vi "read Txt Files.vi"(10 "file path (use dialog)":path) -> (1 "error out":errorcluster, 2 "number":T1)   [LabVIEW 2017] (continued)
Position(0.1mm)¡G\t0.000000\tVelocity(0.1mm0/s)¡G\t0.000000\tVoltage¡G\t-0.009460\nReal Periold(ms)¡G\t1\tEncoder Position(0.1mm)¡G\t0.000000\tVelocity(0.1mm0/s)¡G\t0.000000\tVoltage¡G\t-0.001801\nReal Periold(ms)¡G\t1\tEncoder Position(0.1mm)¡G\t0.000000\tVelocity(0.1mm0/s)¡G\t0.000000\tVoltage¡G\t0.034485\nReal Periold(ms)¡G\t1\tEncoder Position(0.1mm)¡G\t0.000000\tVelocity(0.1mm0/s)¡G\t0.000000\tVoltage¡G\t-0.005951\nReal Periold(ms)¡G\t1\tEncoder Position(0.1mm)¡G\t0.000000\tVelocity(0.1mm0/s)¡G\t0.000000\tVoltage¡G\t0.003601\nReal Periold(ms)¡G\t1\tEncoder Position(0.1mm)¡G\t0.000000\tVelocity(0.1mm0/s)¡G\t0.000000\tVoltage¡G\t0.002319\nReal Periold(ms)¡G\t1\tEncoder Position(0.1mm)¡G\t0.000000\tVelocity(0.1mm0/s)¡G\t0.000000\tVoltage¡G\t0.000092\nReal Periold(ms)¡G\t1\tEncoder Position(0.1mm)¡G\t0.000000\tVelocity(0.1mm0/s)¡G\t0.000000\tVoltage¡G\t0.002960\nReal Periold(ms)¡G\t1\tEncoder Position(0.1mm)¡G\t0.000000\tVelocity(0.1mm0/s)¡G\t0.000000\tVoltage¡G\t0.002319\nReal Periold(ms)¡G\t1\tEncoder Position(0.1mm)¡G\t0.000000\tVelocity(0.1mm0/s)¡G\t0.000000\tVoltage¡G\t0.004883\nReal Periold(ms)¡G\t1\tEncoder Position(0.1mm)¡G\t0.000000\tVelocity(0.1mm0/s)¡G\t0.000000\tVoltage¡G\t-0.004669\nReal Periold(ms)¡G\t1\tEncoder Position(0.1mm)¡G\t0.000000\tVelocity(0.1mm0/s)¡G\t0.000000\tVoltage¡G\t-0.003723\nReal Periold(ms)¡G\t1\tEncoder Position(0.1mm)¡G\t0.000000\tVelocity(0.1mm0/s)¡G\t0.000000\tVoltage¡G\t0.004883\nReal Periold(ms)¡G\t1\tEncoder Position(0.1mm)¡G\t0.000000\tVelocity(0.1mm0/s)¡G\t0.000000\tVoltage¡G\t-0.007843\nReal Periold(ms)¡G\t1\tEncoder Position(0.1mm)¡G\t0.000000\tVelocity(0.1mm0/s)¡G\t0.000000\tVoltage¡G\t-0.005951\nReal Periold(ms)¡G\t1\tEncoder Position(0.1mm)¡G\t0.000000\tVelocity(0.1mm0/s)¡G\t0.000000\tVoltage¡G\t-0.007538\nReal Periold(ms)¡G\t1\tEncoder Position(0.1mm)¡G\t0.000000\tVelocity(0.1mm0/s)¡G\t0.000000\tVoltage¡G\t-0.001495\nReal Periold(ms)¡G\t1\tEncoder Position(0.1mm)¡G\t0.000000\tVelocity(0.1mm0/s)¡G\t0.000000\tVoltage¡G\t-0.001801\nReal Periold(ms)¡G\t1\tEncoder Position(0.1mm)¡G\t0.000000\tVelocity(0.1mm0/s)¡G\t0.000000\tVoltage¡G\t-0.006592\nReal Periold(ms)¡G\t1\tEncoder Position(0.1mm)¡G\t0.000000\tVelocity(0.1mm0/s)¡G\t0.000000\tVoltage¡G\t0.002655\nReal Periold(ms)¡G\t1\tEncoder Position(0.1mm)¡G\t0.000000\tVelocity(0.1mm0/s)¡G\t0.000000\tVoltage¡G\t-0.007843\nReal Periold(ms)¡G\t1\tEncoder Position(0.1mm)¡G\t0.000000\tVelocity(0.1mm0/s)¡G\t0.000000\tVoltage¡G\t-0.007538\nReal Periold(ms)¡G\t1\tEncoder Position(0.1mm)¡G\t0.000000\tVelocity(0.1mm0/s)¡G\t0.000000\tVoltage¡G\t0.006775\nReal Periold(ms)¡G\t1\tEncoder Position(0.1mm)¡G\t0.000000\tVelocity(0.1mm0/s)¡G\t0.000000\tVoltage¡G\t0.005188\nReal Periold(ms)¡G\t1\tEncoder Position(0.1mm)¡G\t0.000000\tVelocity(0.1mm0/s)¡G\t0.000000\tVoltage¡G\t-0.068329\nReal Periold(ms)¡G\t1\tEncoder Position(0.1mm)¡G\t0.000000\tVelocity(0.1mm0/s)¡G\t0.000000\tVoltage¡G\t0.000732\nReal Periold(ms)¡G\t1\tEncoder Position(0.1mm)¡G\t0.000000\tVelocity(0.1mm0/s)¡G\t0.000000\tVoltage¡G\t0.002014\nReal Periold(ms)¡G\t1\tEncoder Position(0.1mm)¡G\t0.000000\tVelocity(0.1mm0/s)¡G\t0.000000\tVoltage¡G\t-0.003082\nReal Periold(ms)¡G\t1\tEncoder Position(0.1mm)¡G\t0.000000\tVelocity(0.1mm0/s)¡G\t0.000000\tVoltage¡G\t-0.022827\nReal Periold(ms)¡G\t1\tEncoder Position(0.1mm)¡G\t0.000000\tVelocity(0.1mm0/s)¡G\t0.000000\tVoltage¡G\t0.007416\nReal Periold(ms)¡G\t1\tEncoder Position(0.1mm)¡G\t0.000000\tVelocity(0.1mm0/s)¡G\t0.000000\tVoltage¡G\t-0.004028\nReal Periold(ms)¡G\t1\tEncoder Position(0.1mm)¡G\t0.000000\tVelocity(0.1mm0/s)¡G\t0.000000\tVoltage¡G\t-0.002441\nReal Periold(ms)¡G\t1\tEncoder Position(0.1mm)¡G\t0.000000\tVelocity(0.1mm0/s)¡G\t0.000000\tVoltage¡G\t-0.001160\nReal Periold(ms)¡G\t1\tEncoder Position(0.1mm)¡G\t0.000000\tVelocity(0.1mm0/s)¡G\t0.000000\tVoltage¡G\t0.000427\nReal Periold(ms)¡G\t1\tEncoder Position(0.1mm)¡G\t0.000000\tVelocity(0.1mm0/s)¡G\t0.000000\tVoltage¡G\t-0.012299\nReal Periold(ms)¡G\t1\tEncoder Position(0.1mm)¡G\t0.000000\tVelocity(0.1mm0/s)¡G\t0.000000\tVoltage¡G\t0.007111\nReal Periold(ms)¡G\t1\tEncoder Position(0.1mm)¡G\t0.000000\tVelocity(0.1mm0/s)¡G\t0.000000\tVoltage¡G\t-0.057831\nReal Periold(ms)¡G\t1\tEncoder Position(0.1mm)¡G\t0.000000\tVelocity(0.1mm0/s)¡G\t0.000000\tVoltage¡G\t0.005524\nReal Periold(ms)¡G\t1\tEncoder Position(0.1mm)¡G\t0.000000\tVelocity(0.1mm0/s)¡G\t0.000000\tVoltage¡G\t-0.004669\nReal Periold(ms)¡G\t1\tEncoder Position(0.1mm)¡G\t0.000000\tVelocity(0.1mm0/s)¡G\t0.000000\tVoltage¡G\t-0.002777\nReal Periold(ms)¡G\t1\tEncoder Position(0.1mm)¡G\t0.000000\tVelocity(0.1mm0/s)¡G\t0.000000\tVoltage¡G\t-0.005005\nReal Periold(ms)¡G\t1\tEncoder Position(0.1mm)¡G\t0.000000\tVelocity(0.1mm0/s)¡G\t0.000000\tVoltage¡G\t-0.005005\nReal Periold(ms)¡G\t1\tEncoder Position(0.1mm)¡G\t0.000000\tVelocity(0.1mm0/s)¡G\t0.000000\tVoltage¡G\t0.010284\nReal Periold(ms)¡G\t1\tEncoder Position(0.1mm)¡G\t0.000000\tVelocity(0.1mm0/s)¡G\t0.000000\tVoltage¡G\t-0.002777\nReal Periold(ms)¡G\t1\tEncoder Position(0.1mm)¡G\t0.000000\tVelocity(0.1mm0/s)¡G\t0.000000\tVoltage¡G\t-0.010071\nReal Periold(ms)¡G\t1\tEncoder Position(0.1mm)¡G\t0.000000\tVelocity(0.1mm0/s)¡G\t0.000000\tVoltage¡G\t0.001373\nReal Periold(ms)¡G\t1\tEncoder Position(0.1mm)¡G\t0.000000\tVelocity(0.1mm0/s)¡G\t0.000000\tVoltage¡G\t-0.001801\nReal Periold(ms)¡G\t1\tEncoder Position(0.1mm)¡G\t0.000000\tVelocity(0.1mm0/s)¡G\t0.000000\tVoltage¡G\t-0.003723\nReal Periold(ms)¡G\t1\tEncoder Position(0.1mm)¡G\t0.000000\tVelocity(0.1mm0/s)¡G\t0.000000\tVoltage¡G\t0.010590\nReal Periold(ms)¡G\t1\tEncoder Position(0.1mm)¡G\t0.000000\tVelocity(0.1mm0/s)¡G\t0.000000\tVoltage¡G\t0.002014\nReal Periold(ms)¡G\t1\tEncoder Position(0.1mm)¡G\t0.000000\tVelocity(0.1mm0/s)¡G\t0.000000\tVoltage¡G\t-0.005310\nReal Periold(ms)¡G\t1\tEncoder Position(0.1mm)¡G\t0.000000\tVelocity(0.1mm0/s)¡G\t0.000000\tVoltage¡G\t0.002655\nReal Periold(ms)¡G\t1\tEncoder Position(0.1mm)¡G\t0.000000\tVelocity(0.1mm0/s)¡G\t0.000000\tVoltage¡G\t-0.011353\nReal Periold(ms)¡G\t1\tEncoder Position(0.1mm)¡G\t0.000000\tVelocity(0.1mm0/s)¡G\t0.000000\tVoltage¡G\t0.001068\nReal Periold(ms)¡G\t1\tEncoder Position(0.1mm)¡G\t0.000000\tVelocity(0.1mm0/s)¡G\t0.000000\tVoltage¡G\t-0.002136\nReal Periold(ms)¡G\t1\tEncoder Position(0.1mm)¡G\t0.000000\tVelocity(0.1mm0/s)¡G\t0.000000\tVoltage¡G\t-0.003387\nReal Periold(ms)¡G\t1\tEncoder Position(0.1mm)¡G\t0.000000\tVelocity(0.1mm0/s)¡G\t0.000000\tVoltage¡G\t0.003601\nReal Periold(ms)¡G\t1\tEncoder Position(0.1mm)¡G\t0.000000\tVelocity(0.1mm0/s)¡G\t0.000000\tVoltage¡G\t0.001068\nReal Periold(ms)¡G\t1\tEncoder Position(0.1mm)¡G\t0.000000\tVelocity(0.1mm0/s)¡G\t0.000000\tVoltage¡G\t-0.005005\nReal Periold(ms)¡G\t1\tEncoder Position(0.1mm)¡G\t0.000000\tVelocity(0.1mm0/s)¡G\t0.000000\tVoltage¡G\t-0.014526\nReal Periold(ms)¡G\t1\tEncoder Position(0.1mm)¡G\t0.000000\tVelocity(0.1mm0/s)¡G\t0.000000\tVoltage¡G\t0.005188\nReal Periold(ms)¡G\t1\tEncoder Position(0.1mm)¡G\t0.000000\tVelocity(0.1mm0/s)¡G\t0.000000\tVoltage¡G\t-0.000214\nReal Periold(ms)¡G\t1\tEncoder Position(0.1mm)¡G\t0.000000\tVelocity(0.1mm0/s)¡G\t0.000000\tVoltage¡G\t-0.002136\nReal Periold(ms)¡G\t1\tEncoder Position(0.1mm)¡G\t0.000000\tVelocity(0.1mm0/s)¡G\t0.000000\tVoltage¡G\t-0.005310\nReal Periold(ms)¡G\t1\tEncoder Position(0.1mm)¡G\t0.000000\tVelocity(0.1mm0/s)¡G\t0.000000\tVoltage¡G\t-0.002777\nReal Periold(ms)¡G\t1\tEncoder Position(0.1mm)¡G\t0.000000\tVelocity(0.1mm0/s)¡G\t0.000000\tVoltage¡G\t0.001373\nReal Periold(ms)¡G\t1\tEncoder Position(0.1mm)¡G\t0.000000\tVelocity(0.1mm0/s)¡G\t0.000000\tVoltage¡G\t-0.013580\nReal Periold(ms)¡G\t1\tEncoder Position(0.1mm)¡G\t0.000000\tVelocity(0.1mm0/s)¡G\t0.000000\tVoltage¡G\t-0.009460\nReal Periold(ms)¡G\t1\tEncoder Position(0.1mm)¡G\t0.000000\tVelocity(0.1mm0/s)¡G\t0.000000\tVoltage¡G\t-0.002441\nReal Periold(ms)¡G\t1\tEncoder Position(0.1mm)¡G\t0.000000\tVelocity(0.1mm0/s)¡G\t0.000000\tVoltage¡G\t0.011230\nReal Periold(ms)¡G\t1\tEncoder Position(0.1mm)¡G\t0.000000\tVelocity(0.1mm0/s)¡G\t0.000000\tVoltage¡G\t-0.005951\nReal Periold(ms)¡G\t1\tEncoder Position(0.1mm)¡G\t0.000000\tVelocity(0.1mm0/s)¡G\t0.000000\tVoltage¡G\t0.008362\nReal Periold(ms)¡G\t1\tEncoder Position(0.1mm)¡G\t0.000000\tVelocity(0.1mm0/s)¡G\t0.000000\tVoltage¡G\t0.009979\nReal Periold(ms)¡G\t1\tEncoder Position(0.1mm)¡G\t0.000000\tVelocity(0.1mm0/s)¡G\t0.000000\tVoltage¡G\t-0.008179\nReal Periold(ms)¡G\t1\tEncoder Position(0.1mm)¡G\t0.000000\tVelocity(0.1mm0/s)¡G\t0.000000\tVoltage¡G\t-0.003723\nReal Periold(ms)¡G\t1\tEncoder Position(0.1mm)¡G\t0.000000\tVelocity(0.1mm0/s)¡G\t0.000000\tVoltage¡G\t0.008362\nReal Periold(ms)¡G\t1\tEncoder Position(0.1mm)¡G\t0.000000\tVelocity(0.1mm0/s)¡G\t0.000000\tVoltage¡G\t-0.001801\nReal Periold(ms)¡G\t1\tEncoder Position(0.1mm)¡G\t0.000000\tVelocity(0.1mm0/s)¡G\t0.000000\tVoltage¡G\t0.000092\nReal Periold(ms)¡G\t1\tEncoder Position(0.1mm)¡G\t0.000000\tVelocity(0.1mm0/s)¡G\t0.000000\tVoltage¡G\t-0.005951\nReal Periold(ms)¡G\t1\tEncoder Position(0.1mm)¡G\t0.000000\tVelocity(0.1mm0/s)¡G\t0.000000\tVoltage¡G\t-0.014221\nReal Periold(ms)¡G\t1\tEncoder Position(0.1mm)¡G\t0.000000\tVelocity(0.1mm0/s)¡G\t0.000000\tVoltage¡G\t-0.005005\nReal Periold(ms)¡G\t1\tEncoder Position(0.1mm)¡G\t0.000000\tVelocity(0.1mm0/s)¡G\t0.000000\tVoltage¡G\t0.050720\nReal Periold(ms)¡G\t1\tEncoder Position(0.1mm)¡G\t0.000000\tVelocity(0.1mm0/s)¡G\t0.000000\tVoltage¡G\t0.006775\nReal Periold(ms)¡G\t1\tEncoder Position(0.1mm)¡G\t0.000000\tVelocity(0.1mm0/s)¡G\t0.000000\tVoltage¡G\t-0.003387\nReal Periold(ms)¡G\t1\tEncoder Position(0.1mm)¡G\t0.000000\tVelocity(0.1mm0/s)¡G\t0.000000\tVoltage¡G\t0.003601\nReal Periold(ms)¡G\t1\tEncoder Position(0.1mm)¡G\t0.000000\tVelocity(0.1mm0/s)¡G\t0.000000\tVoltage¡G\t0.000092\nReal Periold(ms)¡G\t1\tEncoder Position(0.1mm)¡G\t0.000000\tVelocity(0.1mm0/s)¡G\t0.000000\tVoltage¡G\t-0.000854\nReal Periold(ms)¡G\t1\tEncoder Position(0.1mm)¡G\t0.000000\tVelocity(0.1mm0/s)¡G\t0.000000\tVoltage¡G\t-0.004028\nReal Periold(ms)¡G\t1\tEncoder Position(0.1mm)¡G\t0.000000\tVelocity(0.1mm0/s)¡G\t0.000000\tVoltage¡G\t0.000427\nReal Periold(ms)¡G\t1\tEncoder Position(0.1mm)¡G\t0.000000\tVelocity(0.1mm0/s)¡G\t0.000000\tVoltage¡G\t0.002655\nReal Periold(ms)¡G\t1\tEncoder Position(0.1mm)¡G\t0.000000\tVelocity(0.1mm0/s)¡G\t0.000000\tVoltage¡G\t-0.007843\nReal Periold(ms)¡G\t1\tEncoder Position(0.1mm)¡G\t0.000000\tVelocity(0.1mm0/s)¡G\t0.000000\tVoltage¡G\t0.000092\nReal Periold(ms)¡G\t1\tEncoder Position(0.1mm)¡G\t0.000000\tVelocity(0.1mm0/s)¡G\t0.000000\tVoltage¡G\t-0.009125\nReal Periold(ms)¡G\t1\tEncoder Position(0.1mm)¡G\t0.000000\tVelocity(0.1mm0/s)¡G\t0.000000\tVoltage¡G\t0.010284\nReal Periold(ms)¡G\t1\tEncoder Position(0.1mm)¡G\t0.000000\tVelocity(0.1mm0/s)¡G\t0.000000\tVoltage¡G\t0.002960\nReal Periold(ms)¡G\t1\tEncoder Position(0.1mm)¡G\t0.000000\tVelocity(0.1mm0/s)¡G\t0.000000\tVoltage¡G\t0.002960\nReal Periold(ms)¡G\t1\tEncoder Position(0.1mm)¡G\t0.000000\tVelocity(0.1mm0/s)¡G\t0.000000\tVoltage¡G\t0.007751\nReal Periold(ms)¡G\t1\tEncoder Position(0.1mm)¡G\t0.000000\tVelocity(0.1mm0/s)¡G\t0.000000\tVoltage¡G\t0.008057\nReal Periold(ms)¡G\t1\tEncoder Position(0.1mm)¡G\t0.000000\tVelocity(0.1mm0/s)¡G\t0.000000\tVoltage¡G\t-0.000214\nReal Periold(ms)¡G\t1\tEncoder Position(0.1mm)¡G\t0.000000\tVelocity(0.1mm0/s)¡G\t0.000000\tVoltage¡G\t-0.004028\nReal Periold(ms)¡G\t1\tEncoder Position(0.1mm)¡G\t0.000000\tVelocity(0.1mm0/s)¡G\t0.000000\tVoltage¡G\t-0.003723\nReal Periold(ms)¡G\t1\tEncoder Position(0.1mm)¡G\t0.000000\tVelocity(0.1mm0/s)¡G\t0.000000\tVoltage¡G\t-0.002777\nReal Periold(ms)¡G\t1\tEncoder Position(0.1mm)¡G\t0.000000\tVelocity(0.1mm0/s)¡G\t0.000000\tVoltage¡G\t-0.008179\nReal Periold(ms)¡G\t1\tEncoder Position(0.1mm)¡G\t0.000000\tVelocity(0.1mm0/s)¡G\t0.000000\tVoltage¡G\t-0.010712\nReal Periold(ms)¡G\t1\tEncoder Position(0.1mm)¡G\t0.000000\tVelocity(0.1mm0/s)¡G\t0.000000\tVoltage¡G\t-0.002136\nReal Periold(ms)¡G\t1\tEncoder Position(0.1mm)¡G\t0.000000\tVelocity(0.1mm0/s)¡G\t0.000000\tVoltage¡G\t-0.011353\nReal Periold(ms)¡G\t1\tEncoder Position(0.1mm)¡G\t0.000000\tVelocity(0.1mm0/s)¡G\t0.000000\tVoltage¡G\t0.000092\nReal Periold(ms)¡G\t1\tEncoder Position(0.1mm)¡G\t0.000000\tVelocity(0.1mm0/s)¡G\t0.000000\tVoltage¡G\t0.010590\nReal Periold(ms)¡G\t1\tEncoder Position(0.1mm)¡G\t0.000000\tVelocity(0.1mm0/s)¡G\t0.000000\tVoltage¡G\t-0.023773\nReal Periold(ms)¡G\t1\tEncoder Position(0.1mm)¡G\t0.000000\tVelocity(0.1mm0/s)¡G\t0.000000\tVoltage¡G\t-0.005951\nReal Periold(ms)¡G\t1\tEncoder Position(0.1mm)¡G\t0.000000\tVelocity(0.1mm0/s)¡G\t0.000000\tVoltage¡G\t0.005188\nReal Periold(ms)¡G\t1\tEncoder Position(0.1mm)¡G\t0.000000\tVelocity(0.1mm0/s)¡G\t0.000000\tVoltage¡G\t0.000092\nReal Periold(ms)¡G\t1\tEncoder Position(0.1mm)¡G\t0.000000\tVelocity(0.1mm0/s)¡G\t0.000000\tVoltage¡G\t0.010284\nReal Periold(ms)¡G\t1\tEncoder Position(0.1mm)¡G\t0.000000\tVelocity(0.1mm0/s)¡G\t0.000000\tVoltage¡G\t0.004547\nReal Periold(ms)¡G\t1\tEncoder Position(0.1mm)¡G\t0.000000\tVelocity(0.1mm0/s)¡G\t0.000000\tVoltage¡G\t-0.004364\nReal Periold(ms)¡G\t1\tEncoder Position(0.1mm)¡G\t0.000000\tVelocity(0.1mm0/s)¡G\t0.000000\tVoltage¡G\t0.000092\nReal Periold(ms)¡G\t1\tEncoder Position(0.1mm)¡G\t0.000000\tVelocity(0.1mm0/s)¡G\t0.000000\tVoltage¡G\t-0.010071\nReal Periold(ms)¡G\t1\tEncoder Position(0.1mm)¡G\t0.000000\tVelocity(0.1mm0/s)¡G\t0.000000\tVoltage¡G\t-0.002136\nReal Periold(ms)¡G\t1\tEncoder Position(0.1mm)¡G\t0.000000\tVelocity(0.1mm0/s)¡G\t0.000000\tVoltage¡G\t-0.012634\nReal Periold(ms)¡G\t1\tEncoder Position(0.1mm)¡G\t0.000000\tVelocity(0.1mm0/s)¡G\t0.000000\tVoltage¡G\t0.002960\nReal Periold(ms)¡G\t1\tEncoder Position(0.1mm)¡G\t0.000000\tVelocity(0.1mm0/s)¡G\t0.000000\tVoltage¡G\t-0.013275\nReal Periold(ms)¡G\t1\tEncoder Position(0.1mm)¡G\t0.000000\tVelocity(0.1mm0/s)¡G\t0.000000\tVoltage¡G\t-0.007233\nReal Periold(ms)¡G\t1\tEncoder Position(0.1mm)¡G\t0.000000\tVelocity(0.1mm0/s)¡G\t0.000000\tVoltage¡G\t-0.001495\nReal Periold(ms)¡G\t1\tEncoder Position(0.1mm)¡G\t0.000000\tVelocity(0.1mm0/s)¡G\t0.000000\tVoltage¡G\t0.007111\nReal Periold(ms)¡G\t1\tEncoder Position(0.1mm)¡G\t0.000000\tVelocity(0.1mm0/s)¡G\t0.000000\tVoltage¡G\t-0.004364\nReal Periold(ms)¡G\t1\tEncoder Position(0.1mm)¡G\t0.000000\tVelocity(0.1mm0/s)¡G\t0.000000\tVoltage¡G\t0.000092\nReal Periold(ms)¡G\t1\tEncoder Position(0.1mm)¡G\t0.000000\tVelocity(0.1mm0/s)¡G\t0.000000\tVoltage¡G\t0.024292\nReal Periold(ms)¡G\t1\tEncoder Position(0.1mm)¡G\t0.000000\tVelocity(0.1mm0/s)¡G\t0.000000\tVoltage¡G\t-0.019318\nReal Periold(ms)¡G\t1\tEncoder Position(0.1mm)¡G\t0.000000\tVelocity(0.1mm0/s)¡G\t0.000000\tVoltage¡G\t-0.028870\nReal Periold(ms)¡G\t1\tEncoder Position(0.1mm)¡G\t0.000000\tVelocity(0.1mm0/s)¡G\t0.000000\tVoltage¡G\t-0.002441\nReal Periold(ms)¡G\t1\tEncoder Position(0.1mm)¡G\t0.000000\tVelocity(0.1mm0/s)¡G\t0.000000\tVoltage¡G\t-0.003082\nReal Periold(ms)¡G\t1\tEncoder Position(0.1mm)¡G\t0.000000\tVelocity(0.1mm0/s)¡G\t0.000000\tVoltage¡G\t-0.011688\nReal Periold(ms)¡G\t1\tEncoder Position(0.1mm)¡G\t0.000000\tVelocity(0.1mm0/s)¡G\t0.000000\tVoltage¡G\t0.008698\nReal Periold(ms)¡G\t1\tEncoder Position(0.1mm)¡G\t0.000000\tVelocity(0.1mm0/s)¡G\t0.000000\tVoltage¡G\t-0.003082\nReal Periold(ms)¡G\t1\tEncoder Position(0.1mm)¡G\t0.000000\tVelocity(0.1mm0/s)¡G\t0.000000\tVoltage¡G\t0.017914\nReal Periold(ms)¡G\t1\tEncoder Position(0.1mm)¡G\t0.000000\tVelocity(0.1mm0/s)¡G\t0.000000\tVoltage¡G\t-0.018677\nReal Periold(ms)¡G\t1\tEncoder Position(0.1mm)¡G\t0.000000\tVelocity(0.1mm0/s)¡G\t0.000000\tVoltage¡G\t-0.008179\nReal Periold(ms)¡G\t1\tEncoder Position(0.1mm)¡G\t0.000000\tVelocity(0.1mm0/s)¡G\t0.000000\tVoltage¡G\t-0.009766\nReal Periold(ms)¡G\t1\tEncoder Position(0.1mm)¡G\t0.000000\tVelocity(0.1mm0/s)¡G\t0.000000\tVoltage¡G\t-0.004364\nReal Periold(ms)¡G\t1\tEncoder Position(0.1mm)¡G\t0.000000\tVelocity(0.1mm0/s)¡G\t0.000000\tVoltage¡G\t-0.004669\nReal Periold(ms)¡G\t1\tEncoder Position(0.1mm)¡G\t0.000000\tVelocity(0.1mm0/s)¡G\t0.000000\tVoltage¡G\t0.012207\nReal Periold(ms)¡G\t1\tEncoder Position(0.1mm)¡G\t0.000000\tVelocity(0.1mm0/s)¡G\t0.000000\tVoltage¡G\t0.013153\nReal Periold(ms)¡G\t1\tEncoder Position(0.1mm)¡G\t0.000000\tVelocity(0.1mm0/s)¡G\t0.000000\tVoltage¡G\t-0.011993\nReal Periold(ms)¡G\t1\tEncoder Position(0.1mm)¡G\t0.000000\tVelocity(0.1mm0/s)¡G\t0.000000\tVoltage¡G\t0.000092\nReal Periold(ms)¡G\t1\tEncoder Position(0.1mm)¡G\t0.000000\tVelocity(0.1mm0/s)¡G\t0.000000\tVoltage¡G\t-0.009766\nReal Periold(ms)¡G\t1\tEncoder Position(0.1mm)¡G\t0.000000\tVelocity(0.1mm0/s)¡G\t0.000000\tVoltage¡G\t0.005524\nReal Periold(ms)¡G\t1\tEncoder Position(0.1mm)¡G\t0.000000\tVelocity(0.1mm0/s)¡G\t0.000000\tVoltage¡G\t0.001373\nReal Periold(ms)¡G\t1\tEncoder Position(0.1mm)¡G\t0.000000\tVelocity(0.1mm0/s)¡G\t0.000000\tVoltage¡G\t0.000092\nReal Periold(ms)¡G\t1\tEncoder Position(0.1mm)¡G\t0.000000\tVelocity(0.1mm0/s)¡G\t0.000000\tVoltage¡G\t0.027161\nReal Periold(ms)¡G\t1\tEncoder Position(0.1mm)¡G\t0.000000\tVelocity(0.1mm0/s)¡G\t0.000000\tVoltage¡G\t0.004547\nReal Periold(ms)¡G\t1\tEncoder Position(0.1mm)¡G\t0.000000\tVelocity(0.1mm0/s)¡G\t0.000000\tVoltage¡G\t-0.018677\nReal Periold(ms)¡G\t1\tEncoder Position(0.1mm)¡G\t0.000000\tVelocity(0.1mm0/s)¡G\t0.000000\tVoltage¡G\t-0.002777\nReal Periold(ms)¡G\t1\tEncoder Position(0.1mm)¡G\t0.000000\tVelocity(0.1mm0/s)¡G\t0.000000\tVoltage¡G\t-0.018677\nReal Periold(ms)¡G\t1\tEncoder Position(0.1mm)¡G\t0.000000\tVelocity(0.1mm0/s)¡G\t0.000000\tVoltage¡G\t-0.023773\nReal Periold(ms)¡G\t1\tEncoder Position(0.1mm)¡G\t0.000000\tVelocity(0.1mm0/s)¡G\t0.000000\tVoltage¡G\t-0.002777\nReal Periold(ms)¡G\t1\tEncoder Position(0.1mm)¡G\t0.000000\tVelocity(0.1mm0/s)¡G\t0.000000\tVoltage¡G\t0.004547\nReal Periold(ms)¡G\t1\tEncoder Position(0.1mm)¡G\t0.000000\tVelocity(0.1mm0/s)¡G\t0.000000\tVoltage¡G\t0.030670\nReal Periold(ms)¡G\t1\tEncoder Position(0.1mm)¡G\t0.000000\tVelocity(0.1mm0/s)¡G\t0.000000\tVoltage¡G\t0.014099\nReal Periold(ms)¡G\t1\tEncoder Position(0.1mm)¡G\t0.000000\tVelocity(0.1mm0/s)¡G\t0.000000\tVoltage¡G\t-0.005615\nReal Periold(ms)¡G\t1\tEncoder Position(0.1mm)¡G\t0.000000\tVelocity(0.1mm0/s)¡G\t0.000000\tVoltage¡G\t-0.005615\nReal Periold(ms)¡G\t1\tEncoder Position(0.1mm)¡G\t0.000000\tVelocity(0.1mm0/s)¡G\t0.000000\tVoltage¡G\t0.012817\nReal Periold(ms)¡G\t1\tEncoder Position(0.1mm)¡G\t0.000000\tVelocity(0.1mm0/s)¡G\t0.000000\tVoltage¡G\t-0.001160\nReal Periold(ms)¡G\t1\tEncoder Position(0.1mm)¡G\t0.000000\tVelocity(0.1mm0/s)¡G\t0.000000\tVoltage¡G\t0.046265\nReal Periold(ms)¡G\t1\tEncoder Position(0.1mm)¡G\t0.000000\tVelocity(0.1mm0/s)¡G\t0.000000\tVoltage¡G\t-0.007538\nReal Periold(ms)¡G\t1\tEncoder Position(0.1mm)¡G\t0.000000\tVelocity(0.1mm0/s)¡G\t0.000000\tVoltage¡G\t0.003296\nReal Periold(ms)¡G\t1\tEncoder Position(0.1mm)¡G\t0.000000\tVelocity(0.1mm0/s)¡G\t0.000000\tVoltage¡G\t-0.001495\nReal Periold(ms)¡G\t1\tEncoder Position(0.1mm)¡G\t0.000000\tVelocity(0.1mm0/s)¡G\t0.000000\tVoltage¡G\t0.003906\nReal Periold(ms)¡G\t1\tEncoder Position(0.1mm)¡G\t0.000000\tVelocity(0.1mm0/s)¡G\t0.000000\tVoltage¡G\t0.006775\nReal Periold(ms)¡G\t1\tEncoder Position(0.1mm)¡G\t0.000000\tVelocity(0.1mm0/s)¡G\t0.000000\tVoltage¡G\t0.007751\nReal Periold(ms)¡G\t1\tEncoder Position(0.1mm)¡G\t0.000000\tVelocity(0.1mm0/s)¡G\t0.000000\tVoltage¡G\t-0.002777\nReal Periold(ms)¡G\t1\tEncoder Position(0.1mm)¡G\t0.000000\tVelocity(0.1mm0/s)¡G\t0.000000\tVoltage¡G\t0.000732\nReal Periold(ms)¡G\t1\tEncoder Position(0.1mm)¡G\t0.000000\tVelocity(0.1mm0/s)¡G\t0.000000\tVoltage¡G\t-0.000549\nReal Periold(ms)¡G\t1\tEncoder Position(0.1mm)¡G\t0.000000\tVelocity(0.1mm0/s)¡G\t0.000000\tVoltage¡G\t0.004242\nReal Periold(ms)¡G\t1\tEncoder Position(0.1mm)¡G\t0.000000\tVelocity(0.1mm0/s)¡G\t0.000000\tVoltage¡G\t-0.004364\nReal Periold(ms)¡G\t1\tEncoder Position(0.1mm)¡G\t0.000000\tVelocity(0.1mm0/s)¡G\t0.000000\tVoltage¡G\t0.001373\nReal Periold(ms)¡G\t1\tEncoder Position(0.1mm)¡G\t0.000000\tVelocity(0.1mm0/s)¡G\t0.000000\tVoltage¡G\t-0.005005\nReal Periold(ms)¡G\t1\tEncoder Position(0.1mm)¡G\t0.000000\tVelocity(0.1mm0/s)¡G\t0.000000\tVoltage¡G\t0.007416\nReal Periold(ms)¡G\t1\tEncoder Position(0.1mm)¡G\t0.000000\tVelocity(0.1mm0/s)¡G\t0.000000\tVoltage¡G\t-0.000549\nReal Periold(ms)¡G\t1\tEncoder Position(0.1mm)¡G\t0.000000\tVelocity(0.1mm0/s)¡G\t0.000000\tVoltage¡G\t0.018555\nReal Periold(ms)¡G\t1\tEncoder Position(0.1mm)¡G\t0.000000\tVelocity(0.1mm0/s)¡G\t0.000000\tVoltage¡G\t-0.000549\nReal Periold(ms)¡G\t1\tEncoder Position(0.1mm)¡G\t0.000000\tVelocity(0.1mm0/s)¡G\t0.000000\tVoltage¡G\t-0.009766\nReal Periold(ms)¡G\t1\tEncoder Position(0.1mm)¡G\t0.000000\tVelocity(0.1mm0/s)¡G\t0.000000\tVoltage¡G\t-0.005005\nReal Periold(ms)¡G\t1\tEncoder Position(0.1mm)¡G\t0.000000\tVelocity(0.1mm0/s)¡G\t0.000000\tVoltage¡G\t0.001678\nReal Periold(ms)¡G\t1\tEncoder Position(0.1mm)¡G\t0.000000\tVelocity(0.1mm0/s)¡G\t0.000000\tVoltage¡G\t-0.000854\nReal Periold(ms)¡G\t1\tEncoder Position(0.1mm)¡G\t0.000000\tVelocity(0.1mm0/s)¡G\t0.000000\tVoltage¡G\t-0.005310\nReal Periold(ms)¡G\t1\tEncoder Position(0.1mm)¡G\t0.000000\tVelocity(0.1mm0/s)¡G\t0.000000\tVoltage¡G\t-0.005005\nReal Periold(ms)¡G\t1\tEncoder Position(0.1mm)¡G\t0.000000\tVelocity(0.1mm0/s)¡G\t0.000000\tVoltage¡G\t-0.005951\nReal Periold(ms)¡G\t1\tEncoder Position(0.1mm)¡G\t0.000000\tVelocity(0.1mm0/s)¡G\t0.000000\tVoltage¡G\t0.017609\nReal Periold(ms)¡G\t1\tEncoder Position(0.1mm)¡G\t0.000000\tVelocity(0.1mm0/s)¡G\t0.000000\tVoltage¡G\t-0.010071\nReal Periold(ms)¡G\t1\tEncoder Position(0.1mm)¡G\t0.000000\tVelocity(0.1mm0/s)¡G\t0.000000\tVoltage¡G\t0.004883\nReal Periold(ms)¡G\t1\tEncoder Position(0.1mm)¡G\t0.000000\tVelocity(0.1mm0/s)¡G\t0.000000\tVoltage¡G\t-0.001801\nReal Periold(ms)¡G\t1\tEncoder Position(0.1mm)¡G\t0.000000\tVelocity(0.1mm0/s)¡G\t0.000000\tVoltage¡G\t-0.008179\nReal Periold(ms)¡G\t1\tEncoder Position(0.1mm)¡G\t0.000000\tVelocity(0.1mm0/s)¡G\t0.000000\tVoltage¡G\t0.028442\nReal Periold(ms)¡G\t1\tEncoder Position(0.1mm)¡G\t0.000000\tVelocity(0.1mm0/s)¡G\t0.000000\tVoltage¡G\t0.001373\nReal Periold(ms)¡G\t1\tEncoder Position(0.1mm)¡G\t0.000000\tVelocity(0.1mm0/s)¡G\t0.000000\tVoltage¡G\t0.011566\nReal Periold(ms)¡G\t1\tEncoder Position(0.1mm)¡G\t0.000000\tVelocity(0.1mm0/s)¡G\t0.000000\tVoltage¡G\t-0.017395\nReal Periold(ms)¡G\t1\tEncoder Position(0.1mm)¡G\t0.000000\tVelocity(0.1mm0/s)¡G\t0.000000\tVoltage¡G\t-0.009766\nReal Periold(ms)¡G\t1\tEncoder Position(0.1mm)¡G\t0.000000\tVelocity(0.1mm0/s)¡G\t0.000000\tVoltage¡G\t0.003296\nReal Periold(ms)¡G\t1\tEncoder Position(0.1mm)¡G\t0.000000\tVelocity(0.1mm0/s)¡G\t0.000000\tVoltage¡G\t-0.004669\nReal Periold(ms)¡G\t1\tEncoder Position(0.1mm)¡G\t0.000000\tVelocity(0.1mm0/s)¡G\t0.000000\tVoltage¡G\t-0.002441\nReal Periold(ms)¡G\t1\tEncoder Position(0.1mm)¡G\t0.000000\tVelocity(0.1mm0/s)¡G\t0.000000\tVoltage¡G\t-0.000549\nReal Periold(ms)¡G\t1\tEncoder Position(0.1mm)¡G\t0.000000\tVelocity(0.1mm0/s)¡G\t0.000000\tVoltage¡G\t0.003906\nReal Periold(ms)¡G\t1\tEncoder Position(0.1mm)¡G\t0.000000\tVelocity(0.1mm0/s)¡G\t0.000000\tVoltage¡G\t-0.006592\nReal Periold(ms)¡G\t1\tEncoder Position(0.1mm)¡G\t0.000000\tVelocity(0.1mm0/s)¡G\t0.000000\tVoltage¡G\t0.024933\nReal Periold(ms)¡G\t1\tEncoder Position(0.1mm)¡G\t0.000000\tVelocity(0.1mm0/s)¡G\t0.000000\tVoltage¡G\t-0.004669\nReal Periold(ms)¡G\t1\tEncoder Position(0.1mm)¡G\t0.000000\tVelocity(0.1mm0/s)¡G\t0.000000\tVoltage¡G\t-0.006897\nReal Periold(ms)¡G\t1\tEncoder Position(0.1mm)¡G\t0.000000\tVelocity(0.1mm0/s)¡G\t0.000000\tVoltage¡G\t0.002319\nReal Periold(ms)¡G\t1\tEncoder Position(0.1mm)¡G\t0.000000\tVelocity(0.1mm0/s)¡G\t0.000000\tVoltage¡G\t0.002655\nReal Periold(ms)¡G\t1\tEncoder Position(0.1mm)¡G\t0.000000\tVelocity(0.1mm0/s)¡G\t0.000000\tVoltage¡G\t-0.010071\nReal Periold(ms)¡G\t1\tEncoder Position(0.1mm)¡G\t0.000000\tVelocity(0.1mm0/s)¡G\t0.000000\tVoltage¡G\t0.003601\nReal Periold(ms)¡G\t1\tEncoder Position(0.1mm)¡G\t0.000000\tVelocity(0.1mm0/s)¡G\t0.000000\tVoltage¡G\t-0.009460\nReal Periold(ms)¡G\t1\tEncoder Position(0.1mm)¡G\t0.000000\tVelocity(0.1mm0/s)¡G\t0.000000\tVoltage¡G\t-0.000854\nReal Periold(ms)¡G\t1\tEncoder Position(0.1mm)¡G\t0.000000\tVelocity(0.1mm0/s)¡G\t0.000000\tVoltage¡G\t0.005524\nReal Periold(ms)¡G\t1\tEncoder Position(0.1mm)¡G\t0.000000\tVelocity(0.1mm0/s)¡G\t0.000000\tVoltage¡G\t0.007416\nReal Periold(ms)¡G\t1\tEncoder Position(0.1mm)¡G\t0.000000\tVelocity(0.1mm0/s)¡G\t0.000000\tVoltage¡G\t0.005524\nReal Periold(ms)¡G\t1\tEncoder Position(0.1mm)¡G\t0.000000\tVelocity(0.1mm0/s)¡G\t0.000000\tVoltage¡G\t-0.012939\nReal Periold(ms)¡G\t1\tEncoder Position(0.1mm)¡G\t0.000000\tVelocity(0.1mm0/s)¡G\t0.000000\tVoltage¡G\t-0.005310\nReal Periold(ms)¡G\t1\tEncoder Position(0.1mm)¡G\t0.000000\tVelocity(0.1mm0/s)¡G\t0.000000\tVoltage¡G\t-0.008179\nReal Periold(ms)¡G\t1\tEncoder Position(0.1mm)¡G\t0.000000\tVelocity(0.1mm0/s)¡G\t0.000000\tVoltage¡G\t-0.012939\nReal Periold(ms)¡G\t1\tEncoder Position(0.1mm)¡G\t0.000000\tVelocity(0.1mm0/s)¡G\t0.000000\tVoltage¡G\t-0.039368\nReal Periold(ms)¡G\t1\tEncoder Position(0.1mm)¡G\t0.000000\tVelocity(0.1mm0/s)¡G\t0.000000\tVoltage¡G\t-0.005005\nReal Periold(ms)¡G\t1\tEncoder Position(0.1mm)¡G\t0.000000\tVelocity(0.1mm0/s)¡G\t0.000000\tVoltage¡G\t-0.001801\nReal Periold(ms)¡G\t1\tEncoder Position(0.1mm)¡G\t0.000000\tVelocity(0.1mm0/s)¡G\t0.000000\tVoltage¡G\t-0.000854\nReal Periold(ms)¡G\t1\tEncoder Position(0.1mm)¡G\t0.000000\tVelocity(0.1mm0/s)¡G\t0.000000\tVoltage¡G\t-0.001801\nReal Periold(ms)¡G\t1\tEncoder Position(0.1mm)¡G\t0.000000\tVelocity(0.1mm0/s)¡G\t0.000000\tVoltage¡G\t0.007751\nReal Periold(ms)¡G\t1\tEncoder Position(0.1mm)¡G\t0.000000\tVelocity(0.1mm0/s)¡G\t0.000000\tVoltage¡G\t0.007111\nReal Periold(ms)¡G\t1\tEncoder Position(0.1mm)¡G\t0.000000\tVelocity(0.1mm0/s)¡G\t0.000000\tVoltage¡G\t0.007751\nReal Periold(ms)¡G\t1\tEncoder Position(0.1mm)¡G\t0.000000\tVelocity(0.1mm0/s)¡G\t0.000000\tVoltage¡G\t0.003296\nReal Periold(ms)¡G\t1\tEncoder Position(0.1mm)¡G\t0.000000\tVelocity(0.1mm0/s)¡G\t0.000000\tVoltage¡G\t0.001068\nReal Periold(ms)¡G\t1\tEncoder Position(0.1mm)¡G\t0.000000\tVelocity(0.1mm0/s)¡G\t0.000000\tVoltage¡G\t-0.007538\nReal Periold(ms)¡G\t1\tEncoder Position(0.1mm)¡G\t0.000000\tVelocity(0.1mm0/s)¡G\t0.000000\tVoltage¡G\t-0.005005\nReal Periold(ms)¡G\t1\tEncoder Position(0.1mm)¡G\t0.000000\tVelocity(0.1mm0/s)¡G\t0.000000\tVoltage¡G\t0.002960\nReal Periold(ms)¡G\t1\tEncoder Position(0.1mm)¡G\t0.000000\tVelocity(0.1mm0/s)¡G\t0.000000\tVoltage¡G\t0.009644\nReal Periold(ms)¡G\t1\tEncoder Position(0.1mm)¡G\t0.000000\tVelocity(0.1mm0/s)¡G\t0.000000\tVoltage¡G\t0.002014\nReal Periold(ms)¡G\t1\tEncoder Position(0.1mm)¡G\t0.000000\tVelocity(0.1mm0/s)¡G\t0.000000\tVoltage¡G\t0.000427\nReal Periold(ms)¡G\t1\tEncoder Position(0.1mm)¡G\t0.000000\tVelocity(0.1mm0/s)¡G\t0.000000\tVoltage¡G\t0.002014\nReal Periold(ms)¡G\t1\tEncoder Position(0.1mm)¡G\t0.000000\tVelocity(0.1mm0/s)¡G\t0.000000\tVoltage¡G\t0.004883\nReal Periold(ms)¡G\t1\tEncoder Position(0.1mm)¡G\t0.000000\tVelocity(0.1mm0/s)¡G\t0.000000\tVoltage¡G\t0.007751\nReal Periold(ms)¡G\t1\tEncoder Position(0.1mm)¡G\t0.000000\tVelocity(0.1mm0/s)¡G\t0.000000\tVoltage¡G\t0.013458\nReal Periold(ms)¡G\t1\tEncoder Position(0.1mm)¡G\t0.000000\tVelocity(0.1mm0/s)¡G\t0.000000\tVoltage¡G\t0.004242\nReal Periold(ms)¡G\t1\tEncoder Position(0.1mm)¡G\t0.000000\tVelocity(0.1mm0/s)¡G\t0.000000\tVoltage¡G\t-0.015167\nReal Periold(ms)¡G\t1\tEncoder Position(0.1mm)¡G\t0.000000\tVelocity(0.1mm0/s)¡G\t0.000000\tVoltage¡G\t-0.009125\nReal Periold(ms)¡G\t1\tEncoder Position(0.1mm)¡G\t0.000000\tVelocity(0.1mm0/s)¡G\t0.000000\tVoltage¡G\t0.000732\nReal Periold(ms)¡G\t1\tEncoder Position(0.1mm)¡G\t0.000000\tVelocity(0.1mm0/s)¡G\t0.000000\tVoltage¡G\t-0.000549\nReal Periold(ms)¡G\t1\tEncoder Position(0.1mm)¡G\t0.000000\tVelocity(0.1mm0/s)¡G\t0.000000\tVoltage¡G\t-0.000214\nReal Periold(ms)¡G\t1\tEncoder Position(0.1mm)¡G\t0.000000\tVelocity(0.1mm0/s)¡G\t0.000000\tVoltage¡G\t-0.014862\nReal Periold(ms)¡G\t1\tEncoder Position(0.1mm)¡G\t0.000000\tVelocity(0.1mm0/s)¡G\t0.000000\tVoltage¡G\t-0.010071\nReal Periold(ms)¡G\t1\tEncoder Position(0.1mm)¡G\t0.000000\tVelocity(0.1mm0/s)¡G\t0.000000\tVoltage¡G\t0.004883\nReal Periold(ms)¡G\t1\tEncoder Position(0.1mm)¡G\t0.000000\tVelocity(0.1mm0/s)¡G\t0.000000\tVoltage¡G\t-0.005005\nReal Periold(ms)¡G\t1\tEncoder Position(0.1mm)¡G\t0.000000\tVelocity(0.1mm0/s)¡G\t0.000000\tVoltage¡G\t-0.045105\nReal Periold(ms)¡G\t1\tEncoder Position(0.1mm)¡G\t0.000000\tVelocity(0.1mm0/s)¡G\t0.000000\tVoltage¡G\t-0.019318\nReal Periold(ms)¡G\t1\tEncoder Position(0.1mm)¡G\t0.000000\tVelocity(0.1mm0/s)¡G\t0.000000\tVoltage¡G\t0.004547\nReal Periold(ms)¡G\t1\tEncoder Position(0.1mm)¡G\t0.000000\tVelocity(0.1mm0/s)¡G\t0.000000\tVoltage¡G\t0.016327\nReal Periold(ms)¡G\t1\tEncoder Position(0.1mm)¡G\t0.000000\tVelocity(0.1mm0/s)¡G\t0.000000\tVoltage¡G\t0.003906\nReal Periold(ms)¡G\t1\tEncoder Position(0.1mm)¡G\t0.000000\tVelocity(0.1mm0/s)¡G\t0.000000\tVoltage¡G\t-0.003723\nReal Periold(ms)¡G\t1\tEncoder Position(0.1mm)¡G\t0.000000\tVelocity(0.1mm0/s)¡G\t0.000000\tVoltage¡G\t-0.011688\nReal Periold(ms)¡G\t1\tEncoder Position(0.1mm)¡G\t0.000000\tVelocity(0.1mm0/s)¡G\t0.000000\tVoltage¡G\t-0.007538\nReal Periold(ms)¡G\t1\tEncoder Position(0.1mm)¡G\t0.000000\tVelocity(0.1mm0/s)¡G\t0.000000\tVoltage¡G\t0.002014\nReal Periold(ms)¡G\t1\tEncoder Position(0.1mm)¡G\t0.000000\tVelocity(0.1mm0/s)¡G\t0.000000\tVoltage¡G\t0.003296\nReal Periold(ms)¡G\t1\tEncoder Position(0.1mm)¡G\t0.000000\tVelocity(0.1mm0/s)¡G\t0.000000\tVoltage¡G\t-0.007538\nReal Periold(ms)¡G\t1\tEncoder Position(0.1mm)¡G\t0.000000\tVelocity(0.1mm0/s)¡G\t0.000000\tVoltage¡G\t-0.004028\nReal Periold(ms)¡G\t1\tEncoder Position(0.1mm)¡G\t0.000000\tVelocity(0.1mm0/s)¡G\t0.000000\tVoltage¡G\t-0.008484\nReal Periold(ms)¡G\t1\tEncoder Position(0.1mm)¡G\t0.000000\tVelocity(0.1mm0/s)¡G\t0.000000\tVoltage¡G\t0.019196\nReal Periold(ms)¡G\t1\tEncoder Position(0.1mm)¡G\t0.000000\tVelocity(0.1mm0/s)¡G\t0.000000\tVoltage¡G\t0.002960\nReal Periold(ms)¡G\t1\tEncoder Position(0.1mm)¡G\t0.000000\tVelocity(0.1mm0/s)¡G\t0.000000\tVoltage¡G\t0.004883\nReal Periold(ms)¡G\t1\tEncoder Position(0.1mm)¡G\t0.000000\tVelocity(0.1mm0/s)¡G\t0.000000\tVoltage¡G\t-0.002136\nReal Periold(ms)¡G\t1\tEncoder Position(0.1mm)¡G\t0.000000\tVelocity(0.1mm0/s)¡G\t0.000000\tVoltage¡G\t-0.005951\nReal Periold(ms)¡G\t1\tEncoder Position(0.1mm)¡G\t0.000000\tVelocity(0.1mm0/s)¡G\t0.000000\tVoltage¡G\t-0.005005\nReal Periold(ms)¡G\t1\tEncoder Position(0.1mm)¡G\t0.000000\tVelocity(0.1mm0/s)¡G\t0.000000\tVoltage¡G\t0.003296\nReal Periold(ms)¡G\t1\tEncoder Position(0.1mm)¡G\t0.000000\tVelocity(0.1mm0/s)¡G\t0.000000\tVoltage¡G\t-0.015167\nReal Periold(ms)¡G\t1\tEncoder Position(0.1mm)¡G\t0.000000\tVelocity(0.1mm0/s)¡G\t0.000000\tVoltage¡G\t-0.009460\nReal Periold(ms)¡G\t1\tEncoder Position(0.1mm)¡G\t0.000000\tVelocity(0.1mm0/s)¡G\t0.000000\tVoltage¡G\t-0.013916\nReal Periold(ms)¡G\t1\tEncoder Position(0.1mm)¡G\t0.000000\tVelocity(0.1mm0/s)¡G\t0.000000\tVoltage¡G\t0.005524\nReal Periold(ms)¡G\t1\tEncoder Position(0.1mm)¡G\t0.000000\tVelocity(0.1mm0/s)¡G\t0.000000\tVoltage¡G\t-0.007233\nReal Periold(ms)¡G\t1\tEncoder Position(0.1mm)¡G\t0.000000\tVelocity(0.1mm0/s)¡G\t0.000000\tVoltage¡G\t-0.008484\nReal Periold(ms)¡G\t1\tEncoder Position(0.1mm)¡G\t0.000000\tVelocity(0.1mm0/s)¡G\t0.000000\tVoltage¡G\t0.001373\nReal Periold(ms)¡G\t1\tEncoder Position(0.1mm)¡G\t0.000000\tVelocity(0.1mm0/s)¡G\t0.000000\tVoltage¡G\t-0.000854\nReal Periold(ms)¡G\t1\tEncoder Position(0.1mm)¡G\t0.000000\tVelocity(0.1mm0/s)¡G\t0.000000\tVoltage¡G\t0.007111\nReal Periold(ms)¡G\t1\tEncoder Position(0.1mm)¡G\t0.000000\tVelocity(0.1mm0/s)¡G\t0.000000\tVoltage¡G\t0.007111\nReal Periold(ms)¡G\t1\tEncoder Position(0.1mm)¡G\t0.000000\tVelocity(0.1mm0/s)¡G\t0.000000\tVoltage¡G\t0.003601\nReal Periold(ms)¡G\t1\tEncoder Position(0.1mm)¡G\t0.000000\tVelocity(0.1mm0/s)¡G\t0.000000\tVoltage¡G\t-0.007843\nReal Periold(ms)¡G\t1\tEncoder Position(0.1mm)¡G\t0.000000\tVelocity(0.1mm0/s)¡G\t0.000000\tVoltage¡G\t-0.008820\nReal Periold(ms)¡G\t1\tEncoder Position(0.1mm)¡G\t0.000000\tVelocity(0.1mm0/s)¡G\t0.000000\tVoltage¡G\t-0.003082\nReal Periold(ms)¡G\t1\tEncoder Position(0.1mm)¡G\t0.000000\tVelocity(0.1mm0/s)¡G\t0.000000\tVoltage¡G\t0.009003\nReal Periold(ms)¡G\t1\tEncoder Position(0.1mm)¡G\t0.000000\tVelocity(0.1mm0/s)¡G\t0.000000\tVoltage¡G\t-0.008484\nReal Periold(ms)¡G\t1\tEncoder Position(0.1mm)¡G\t0.000000\tVelocity(0.1mm0/s)¡G\t0.000000\tVoltage¡G\t0.001373\nReal Periold(ms)¡G\t1\tEncoder Position(0.1mm)¡G\t0.000000\tVelocity(0.1mm0/s)¡G\t0.000000\tVoltage¡G\t-0.006897\nReal Periold(ms)¡G\t1\tEncoder Position(0.1mm)¡G\t0.000000\tVelocity(0.1mm0/s)¡G\t0.000000\tVoltage¡G\t0.001678\nReal Periold(ms)¡G\t1\tEncoder Position(0.1mm)¡G\t0.000000\tVelocity(0.1mm0/s)¡G\t0.000000\tVoltage¡G\t0.009003\nReal Periold(ms)¡G\t1\tEncoder Position(0.1mm)¡G\t0.000000\tVelocity(0.1mm0/s)¡G\t0.000000\tVoltage¡G\t0.003296\nReal Periold(ms)¡G\t1\tEncoder Position(0.1mm)¡G\t0.000000\tVelocity(0.1mm0/s)¡G\t0.000000\tVoltage¡G\t0.001373\nReal Periold(ms)¡G\t1\tEncoder Position(0.1mm)¡G\t0.000000\tVelocity(0.1mm0/s)¡G\t0.000000\tVoltage¡G\t0.001373\nReal Periold(ms)¡G\t1\tEncoder Position(0.1mm)¡G\t0.000000\tVelocity(0.1mm0/s)¡G\t0.000000\tVoltage¡G\t-0.002777\nReal Periold(ms)¡G\t1\tEncoder Position(0.1mm)¡G\t0.000000\tVelocity(0.1mm0/s)¡G\t0.000000\tVoltage¡G\t0.009644\nReal Periold(ms)¡G\t1\tEncoder Position(0.1mm)¡G\t0.000000\tVelocity(0.1mm0/s)¡G\t0.000000\tVoltage¡G\t0.015381\nReal Periold(ms)¡G\t1\tEncoder Position(0.1mm)¡G\t0.000000\tVelocity(0.1mm0/s)¡G\t0.000000\tVoltage¡G\t-0.006592\nReal Periold(ms)¡G\t1\tEncoder Position(0.1mm)¡G\t0.000000\tVelocity(0.1mm0/s)¡G\t0.000000\tVoltage¡G\t-0.003387\nReal Periold(ms)¡G\t1\tEncoder Position(0.1mm)¡G\t0.000000\tVelocity(0.1mm0/s)¡G\t0.000000\tVoltage¡G\t-0.005615\nReal Periold(ms)¡G\t1\tEncoder Position(0.1mm)¡G\t0.000000\tVelocity(0.1mm0/s)¡G\t0.000000\tVoltage¡G\t-0.006592\nReal Periold(ms)¡G\t1\tEncoder Position(0.1mm)¡G\t0.000000\tVelocity(0.1mm0/s)¡G\t0.000000\tVoltage¡G\t0.003906\nReal Periold(ms)¡G\t1\tEncoder Position(0.1mm)¡G\t0.000000\tVelocity(0.1mm0/s)¡G\t0.000000\tVoltage¡G\t0.002014\nReal Periold(ms)¡G\t1\tEncoder Position(0.1mm)¡G\t0.000000\tVelocity(0.1mm0/s)¡G\t0.000000\tVoltage¡G\t-0.002441\nReal Periold(ms)¡G\t1\tEncoder Position(0.1mm)¡G\t0.000000\tVelocity(0.1mm0/s)¡G\t0.000000\tVoltage¡G\t-0.005951\nReal Periold(ms)¡G\t1\tEncoder Position(0.1mm)¡G\t0.000000\tVelocity(0.1mm0/s)¡G\t0.000000\tVoltage¡G\t0.000427\nReal Periold(ms)¡G\t1\tEncoder Position(0.1mm)¡G\t0.000000\tVelocity(0.1mm0/s)¡G\t0.000000\tVoltage¡G\t0.008362\nReal Periold(ms)¡G\t1\tEncoder Position(0.1mm)¡G\t0.000000\tVelocity(0.1mm0/s)¡G\t0.000000\tVoltage¡G\t0.007111\nReal Periold(ms)¡G\t1\tEncoder Position(0.1mm)¡G\t0.000000\tVelocity(0.1mm0/s)¡G\t0.000000\tVoltage¡G\t0.078705\nReal Periold(ms)¡G\t1\tEncoder Position(0.1mm)¡G\t0.000000\tVelocity(0.1mm0/s)¡G\t0.000000\tVoltage¡G\t-0.005005\nReal Periold(ms)¡G\t1\tEncoder Position(0.1mm)¡G\t0.000000\tVelocity(0.1mm0/s)¡G\t0.000000\tVoltage¡G\t0.000732\nReal Periold(ms)¡G\t1\tEncoder Position(0.1mm)¡G\t0.000000\tVelocity(0.1mm0/s)¡G\t0.000000\tVoltage¡G\t-0.020264\nReal Periold(ms)¡G\t1\tEncoder Position(0.1mm)¡G\t0.000000\tVelocity(0.1mm0/s)¡G\t0.000000\tVoltage¡G\t0.002319\nReal Periold(ms)¡G\t1\tEncoder Position(0.1mm)¡G\t0.000000\tVelocity(0.1mm0/s)¡G\t0.000000\tVoltage¡G\t-0.003723\nReal Periold(ms)¡G\t1\tEncoder Position(0.1mm)¡G\t0.000000\tVelocity(0.1mm0/s)¡G\t0.000000\tVoltage¡G\t-0.001160\nReal Periold(ms)¡G\t1\tEncoder Position(0.1mm)¡G\t0.000000\tVelocity(0.1mm0/s)¡G\t0.000000\tVoltage¡G\t0.001068\nReal Periold(ms)¡G\t1\tEncoder Position(0.1mm)¡G\t0.000000\tVelocity(0.1mm0/s)¡G\t0.000000\tVoltage¡G\t0.002014\nReal Periold(ms)¡G\t1\tEncoder Position(0.1mm)¡G\t0.000000\tVelocity(0.1mm0/s)¡G\t0.000000\tVoltage¡G\t0.002014\nReal Periold(ms)¡G\t1\tEncoder Position(0.1mm)¡G\t0.000000\tVelocity(0.1mm0/s)¡G\t0.000000\tVoltage¡G\t0.017914\nReal Periold(ms)¡G\t1\tEncoder Position(0.1mm)¡G\t0.000000\tVelocity(0.1mm0/s)¡G\t0.000000\tVoltage¡G\t0.014740\nReal Periold(ms)¡G\t1\tEncoder Position(0.1mm)¡G\t0.000000\tVelocity(0.1mm0/s)¡G\t0.000000\tVoltage¡G\t0.007751\nReal Periold(ms)¡G\t1\tEncoder Position(0.1mm)¡G\t0.000000\tVelocity(0.1mm0/s)¡G\t0.000000\tVoltage¡G\t-0.002136\nReal Periold(ms)¡G\t1\tEncoder Position(0.1mm)¡G\t0.000000\tVelocity(0.1mm0/s)¡G\t0.000000\tVoltage¡G\t-0.006256\nReal Periold(ms)¡G\t1\tEncoder Position(0.1mm)¡G\t0.000000\tVelocity(0.1mm0/s)¡G\t0.000000\tVoltage¡G\t-0.009125\nReal Periold(ms)¡G\t1\tEncoder Position(0.1mm)¡G\t0.000000\tVelocity(0.1mm0/s)¡G\t0.000000\tVoltage¡G\t0.003601\nReal Periold(ms)¡G\t1\tEncoder Position(0.1mm)¡G\t0.000000\tVelocity(0.1mm0/s)¡G\t0.000000\tVoltage¡G\t-0.021240\nReal Periold(ms)¡G\t1\tEncoder Position(0.1mm)¡G\t0.000000\tVelocity(0.1mm0/s)¡G\t0.000000\tVoltage¡G\t-0.007843\nReal Periold(ms)¡G\t1\tEncoder Position(0.1mm)¡G\t0.000000\tVelocity(0.1mm0/s)¡G\t0.000000\tVoltage¡G\t0.006775\nReal Periold(ms)¡G\t1\tEncoder Position(0.1mm)¡G\t0.000000\tVelocity(0.1mm0/s)¡G\t0.000000\tVoltage¡G\t-0.001495\nReal Periold(ms)¡G\t1\tEncoder Position(0.1mm)¡G\t0.000000\tVelocity(0.1mm0/s)¡G\t0.000000\tVoltage¡G\t0.010284\nReal Periold(ms)¡G\t1\tEncoder Position(0.1mm)¡G\t0.000000\tVelocity(0.1mm0/s)¡G\t0.000000\tVoltage¡G\t-0.002777\nReal Periold(ms)¡G\t1\tEncoder Position(0.1mm)¡G\t0.000000\tVelocity(0.1mm0/s)¡G\t0.000000\tVoltage¡G\t0.012817\nReal Periold(ms)¡G\t1\tEncoder Position(0.1mm)¡G\t0.000000\tVelocity(0.1mm0/s)¡G\t0.000000\tVoltage¡G\t0.005188\nReal Periold(ms)¡G\t1\tEncoder Position(0.1mm)¡G\t0.000000\tVelocity(0.1mm0/s)¡G\t0.000000\tVoltage¡G\t0.002014\nReal Periold(ms)¡G\t1\tEncoder Position(0.1mm)¡G\t0.000000\tVelocity(0.1mm0/s)¡G\t0.000000\tVoltage¡G\t0.010590\nReal Periold(ms)¡G\t1\tEncoder Position(0.1mm)¡G\t0.000000\tVelocity(0.1mm0/s)¡G\t0.000000\tVoltage¡G\t0.009979\nReal Periold(ms)¡G\t1\tEncoder Position(0.1mm)¡G\t0.000000\tVelocity(0.1mm0/s)¡G\t0.000000\tVoltage¡G\t-0.003723\nReal Periold(ms)¡G\t1\tEncoder Position(0.1mm)¡G\t0.000000\tVelocity(0.1mm0/s)¡G\t0.000000\tVoltage¡G\t-0.007233\nReal Periold(ms)¡G\t1\tEncoder Position(0.1mm)¡G\t0.000000\tVelocity(0.1mm0/s)¡G\t0.000000\tVoltage¡G\t-0.003723\nReal Periold(ms)¡G\t1\tEncoder Position(0.1mm)¡G\t0.000000\tVelocity(0.1mm0/s)¡G\t0.000000\tVoltage¡G\t-0.000549\nReal Periold(ms)¡G\t1\tEncoder Position(0.1mm)¡G\t0.000000\tVelocity(0.1mm0/s)¡G\t0.000000\tVoltage¡G\t0.002960\nReal Periold(ms)¡G\t1\tEncoder Position(0.1mm)¡G\t0.000000\tVelocity(0.1mm0/s)¡G\t0.000000\tVoltage¡G\t-0.017731\nReal Periold(ms)¡G\t1\tEncoder Position(0.1mm)¡G\t0.000000\tVelocity(0.1mm0/s)¡G\t0.000000\tVoltage¡G\t-0.001801\nReal Periold(ms)¡G\t1\tEncoder Position(0.1mm)¡G\t0.000000\tVelocity(0.1mm0/s)¡G\t0.000000\tVoltage¡G\t-0.001160\nReal Periold(ms)¡G\t1\tEncoder Position(0.1mm)¡G\t0.000000\tVelocity(0.1mm0/s)¡G\t0.000000\tVoltage¡G\t0.002960\nReal Periold(ms)¡G\t1\tEncoder Position(0.1mm)¡G\t0.000000\tVelocity(0.1mm0/s)¡G\t0.000000\tVoltage¡G\t-0.001801\nReal Periold(ms)¡G\t1\tEncoder Position(0.1mm)¡G\t0.000000\tVelocity(0.1mm0/s)¡G\t0.000000\tVoltage¡G\t0.002319\nReal Periold(ms)¡G\t1\tEncoder Position(0.1mm)¡G\t0.000000\tVelocity(0.1mm0/s)¡G\t0.000000\tVoltage¡G\t-0.008820\nReal Periold(ms)¡G\t1\tEncoder Position(0.1mm)¡G\t0.000000\tVelocity(0.1mm0/s)¡G\t0.000000\tVoltage¡G\t-0.003723\nReal Periold(ms)¡G\t1\tEncoder Position(0.1mm)¡G\t0.000000\tVelocity(0.1mm0/s)¡G\t0.000000\tVoltage¡G\t-0.014526\nReal Periold(ms)¡G\t1\tEncoder Position(0.1mm)¡G\t0.000000\tVelocity(0.1mm0/s)¡G\t0.000000\tVoltage¡G\t0.001068\nReal Periold(ms)¡G\t1\tEncoder Position(0.1mm)¡G\t0.000000\tVelocity(0.1mm0/s)¡G\t0.000000\tVoltage¡G\t-0.003082\nReal Periold(ms)¡G\t1\tEncoder Position(0.1mm)¡G\t0.000000\tVelocity(0.1mm0/s)¡G\t0.000000\tVoltage¡G\t-0.060699\nReal Periold(ms)¡G\t1\tEncoder Position(0.1mm)¡G\t0.000000\tVelocity(0.1mm0/s)¡G\t0.000000\tVoltage¡G\t0.014435\nReal Periold(ms)¡G\t1\tEncoder Position(0.1mm)¡G\t0.000000\t
